vi "String Matches Pattern.vi"(10 "Pattern":string="Motors/Left", 11 "Names":string[](array[string])=["/Motors/Left", "/Motors/Right", "/Motors/Shoulder", "/Motors/Elbow", "/Motors/Wrist", "/Solenoid/A", "/Solenoid/B"]) -> (3 "Matching":bool[](array[boolean]))   [LabVIEW 2017]
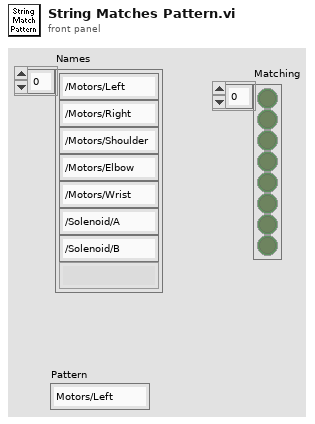
[diagram p1: front panel]
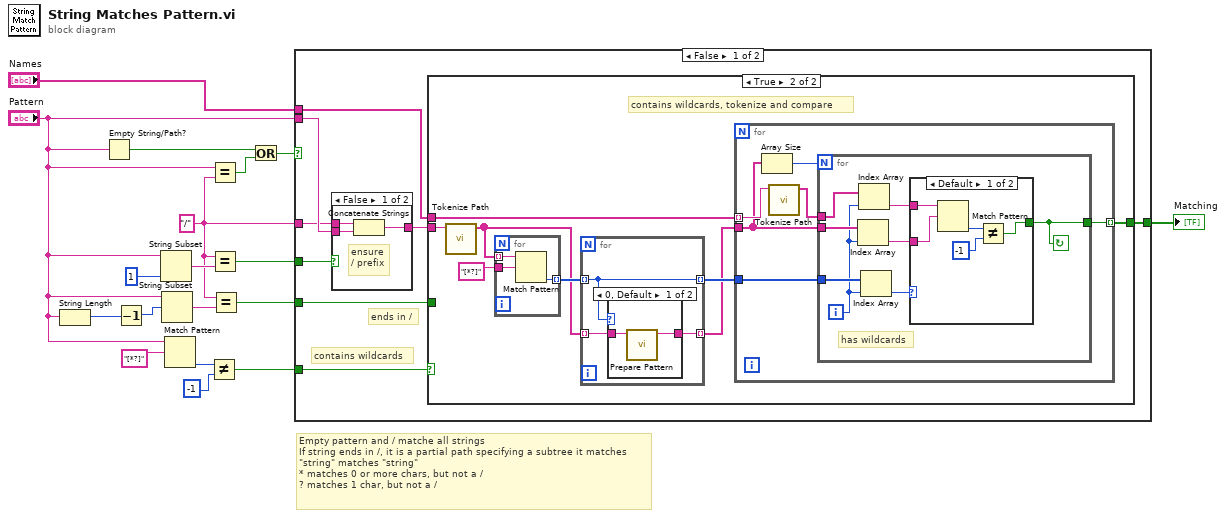
[diagram p0: block diagram]
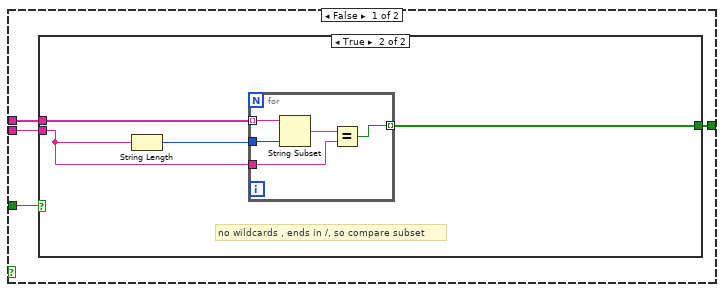
[diagram p2: hidden frame]
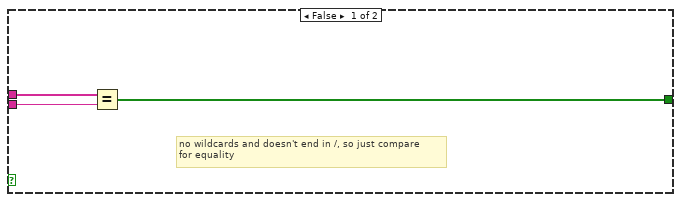
[diagram p3: hidden frame]
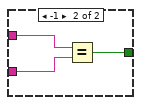
[diagram p5: hidden frame]
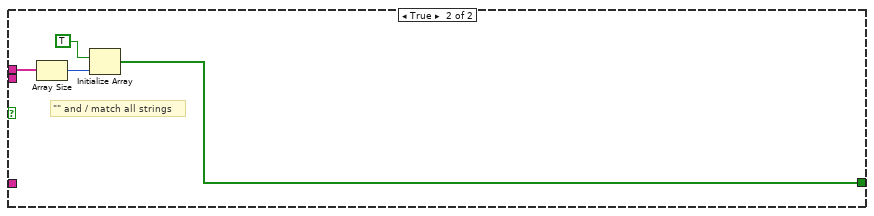
[diagram p7: hidden frame]
diagram:
  w8 = "/"
  # "Empty pattern and / matche all strings\nIf string ends in /, it is a partial path specifying a subtree it matches\n\"string\" matches \"string\"\n* matches 0 or more chars, but not a /\n? matches 1 char, but not a /"
  n1 = String Length(string="Pattern") -> (length=w2:i32)
  n2 = Empty String/Path?(string/path="Pattern") -> (empty?=w9:bool)
  n3 = Decrement(x=w2) -> (x-1=w13:i32)
  n4 = String Subset(string="Pattern", length (rest)=1 ("length (rest)")) -> (substring=w16:string)  [unwired: 1 in]
  n5 = String Subset(string="Pattern", offset (0)=w13) -> (substring=w14:string)  [unwired: 1 in]
  n6 = Match Pattern(string="Pattern", regular expression="[*?]") -> (offset past match=w5:i32)  [unwired: 1 in, 3 out]
  n7 = Not Equal?(x=w5, y=-1 ("length (rest)")) -> (x != y?=w3:bool)
  n8 = Equal?(x="Pattern", y=w8) -> (x = y?=w10:bool)
  n9 = Equal?(x=w8, y=w16) -> (x = y?=w12:bool)
  n10 = Equal?(x=w8, y=w14) -> (x = y?=w7:bool)
  n11 = Or(x=w9, y=w10) -> (x .or. y?=w11:bool)
  n12 = case shown="False" w11 {
    tunnel: [w19 w86] -> w18
    tunnel: "Names" -> [w20 w88]
    tunnel: "Pattern" -> [w26 _]
    tunnel: w8 -> [w25 _]
    tunnel: w12 -> [w24 _]
    tunnel: w7 -> [w21 _]
    tunnel: w3 -> [w22 _]
    frame False {
      # "contains wildcards"
      # "ends in /"
      n13 = case shown="False" w24 {
        tunnel: w25 -> [w84 _]
        tunnel: w26 -> [w83 w85]
        tunnel: [w82 w85] -> w23
        frame False {
          # "ensure\n/ prefix"
          n14 = Concatenate Strings(w84, w83) -> (w82:string)
        }
        frame True {
        }
      }
      n15 = case shown="True" w22 {
        tunnel: w23 -> [w29 w50]
        tunnel: w21 -> [w30 _]
        tunnel: w20 -> [w28 w49]
        tunnel: [w27 w47] -> w19
        frame False {
          n16 = case shown="True" w30 {
            tunnel: w29 -> [w33 w35]
            tunnel: w28 -> [w32 w37]
            tunnel: [w31 w34] -> w27
            frame False {
              # "no wildcards and doesn't end in /, so just compare\nfor equality"
              n17 = Equal?(x=w32, y=w33) -> (x = y?=w31:bool[])
            }
            frame True {
              # "no wildcards , ends in /, so compare subset"
              n18 = String Length(string=w35) -> (length=w36:i32)
              n19 = for {
                tunnel: w37 -> [w42] mode=indexing
                tunnel: w36 -> [w41]
                tunnel: w35 -> [w39]
                tunnel: [w38] -> w34 mode=indexing
                n20 = String Subset(string=w42, length (rest)=w41) -> (substring=w40:string)  [unwired: 1 in]
                n21 = Equal?(x=w40, y=w39) -> (x = y?=w38:bool)
              }
            }
          }
        }
        frame True {
          # "contains wildcards, tokenize and compare"
          n22 = call <vilib>:"Tokenize Path.vi"("Name"=w50) -> ("Array"=w44:string[])  [unwired: 10 in]
          n23 = for {
            tunnel: w44 -> [w59] mode=indexing
            tunnel: "[*?]" -> [w58]
            tunnel: [w57] -> w45 mode=indexing
            n24 = Match Pattern(string=w59, regular expression=w58) -> (offset past match=w57:i32)  [unwired: 1 in, 3 out]
          }
          n25 = for {
            tunnel: [w52] -> w46 mode=indexing
            tunnel: w45 -> [w52] mode=indexing
            tunnel: w44 -> [w53] mode=indexing
            tunnel: [w51] -> w43 mode=indexing
            n26 = case shown="0, Default" w52 {
              tunnel: w53 -> [w55 w56]
              tunnel: [w54 w56] -> w51
              frame 0, Default {
                n27 = call <vilib>:"Prepare Pattern.vi"("Pattern"=w55) -> ("Prepared Pattern"=w54:string)  [unwired: 10 in]
              }
              frame -1 {
              }
            }
          }
          n28 = for {
            tunnel: w43 -> [w63]
            tunnel: w49 -> [w65] mode=indexing
            tunnel: w46 -> [w61]
            tunnel: [w60] -> w47 mode=indexing
            n29 = Array Size(array=w63) -> (size(s)=w62:i32)
            n30 = call <vilib>:"Tokenize Path.vi"("Name"=w65) -> ("Array"=w64:string[])  [unwired: 10 in]
            n31 = for {
              N: w62 -> [_]
              tunnel: w63 -> [w73]
              tunnel: w64 -> [w72]
              tunnel: w61 -> [w69]
              tunnel: [w67] -> w60
              i -> [w66]
              stop <- w67 continue-if-true
              # "has wildcards"
              n32 = Index Array(array=w73, index=w66) -> (element=w70:string)
              n33 = Index Array(array=w72, index=w66) -> (element=w71:string)
              n34 = Index Array(array=w69, index=w66) -> (element=w68:i32)
              n35 = case shown="Default" w68 {
                tunnel: w71 -> [w78 w81]
                tunnel: w70 -> [w74 w80]
                tunnel: [w75 w79] -> w67
                frame Default {
                  n36 = Match Pattern(string=w78, regular expression=w74) -> (offset past match=w77:i32)  [unwired: 1 in, 3 out]
                  n37 = Not Equal?(x=w77, y=-1 ("length (rest)")) -> (x != y?=w75:bool)
                }
                frame -1 {
                  n38 = Equal?(x=w81, y=w80) -> (x = y?=w79:bool)
                }
              }
            }
          }
        }
      }
    }
    frame True {
      # "\"\" and / match all strings"
      n39 = Array Size(array=w88) -> (size(s)=w87:i32)
      n40 = Initialize Array(TRUE, w87) -> (w86:bool[])
    }
  }
  "Matching" <- w18
